vi "属性节点控制界面.vi"() -> ()   [LabVIEW 2010]
panel:
  out "执行:状态":T1(ring)
  out "前面板窗口:状态":T2(ring)
  in  "停止 3":bool
  out "数字(0-1) 3":dbl
  out "前面板窗口:在最前 2":bool
  out "数字(0-1)":dbl
  in  "布尔":bool
  out "2":dbl format="%#_11g"
  in  "停止":bool
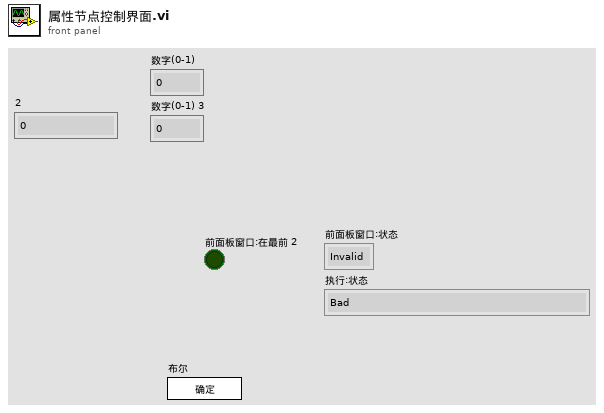
[diagram p1: front panel]
types:
  T1 = enum32{"Bad", "Idle", "Run top level", "Running"}
  T2 = enum32{"Invalid", "Standard", "Closed", "Hidden", "Minimized", "Maximized"}
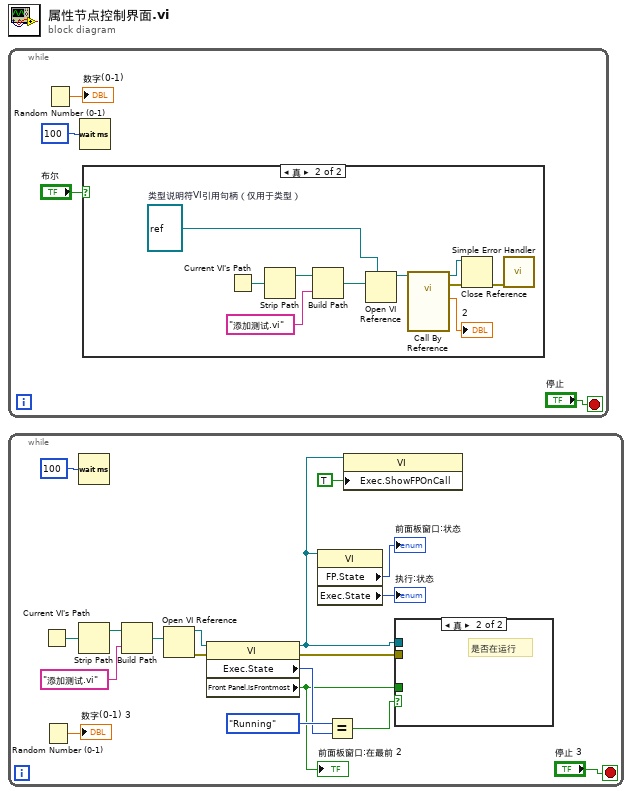
[diagram p0: block diagram]
diagram:
  n1 = while {
    stop <- "停止" stop-if-true
    n2 = Random Number (0-1)() -> (number: 0 to 1=→"数字(0-1)":dbl)
    n3 = Wait (ms)(milliseconds to wait=u32 100 ("等待时间（毫秒）")) -> ()  [unwired: 1 out]
    n4 = case shown="真" "布尔" {
      frame False {
      }
      frame True {
        w9 = refnum<vi> refnum  # 类型说明符VI引用句柄（仅用于类型）
        n5 = Current VI's Path() -> (path=w14:path)
        n6 = Strip Path(path=w14) -> (stripped path=w13:path)  [unwired: 1 out]
        n7 = Build Path(base path=w13, name or relative path="添加测试.vi" ("名称或相对路径")) -> (appended path=w11:path)
        n8 = Open VI Reference(type specifier VI Refnum (for type only)=w9, vi path=w11) -> (vi reference=w10:refnum<vi>)  [unwired: 4 in, 1 out]
        n9 = call-by-ref "?"(reference=w10) -> (reference out=w7:refnum<vi>, error out=w6:errorcluster, "手机号码"=→"2":dbl)  [unwired: 12 in]
        n10 = Close Reference(reference=w7, error in (no error)=w6) -> (error out=w5:errorcluster)
        n11 = call <vilib>:"Simple Error Handler.vi"("error in (no error)"=w5) -> ()  [unwired: 4 in, 5 out]
      }
    }
  }
  n12 = while {
    stop <- "停止 3" stop-if-true
    n13 = Current VI's Path() -> (path=w30:path)
    n14 = Random Number (0-1)() -> (number: 0 to 1=→"数字(0-1) 3":dbl)
    n15 = Wait (ms)(milliseconds to wait=u32 100 ("等待时间（毫秒）")) -> ()  [unwired: 1 out]
    n16 = Strip Path(path=w30) -> (stripped path=w22:path)  [unwired: 1 out]
    n17 = Build Path(base path=w22, name or relative path="添加测试.vi" ("名称或相对路径")) -> (appended path=w20:path)
    n18 = Open VI Reference(vi path=w20) -> (vi reference=w23:refnum<vi>, error out=w24:errorcluster)  [unwired: 5 in]
    n19 = property class="VI"(reference=w23, error in=w24) -> (reference out=w17:refnum<vi>, error out=w26:errorcluster, "Exec.State"=w27:T1, "Front Panel.IsFrontmost"=w25:bool)
    "前面板窗口:在最前 2" <- w25
    n20 = property class="VI"(reference=w17) -> ("FP.State"=→"前面板窗口:状态":T2, "Exec.State"=→"执行:状态":T1)  [unwired: 1 in, 2 out]
    n21 = Equal?(x=T1."Running", y=w27) -> (x = y?=w29:bool)
    n22 = property class="VI"(reference=w17, "Exec.ShowFPOnCall"=TRUE ("执行:调用时显示前面板")) -> ()  [unwired: 1 in, 2 out]
    n23 = case shown="真" w29 {
      tunnel: w25 -> [_ _]
      tunnel: w17 -> [_ _]
      tunnel: w26 -> [_ _]
      frame False {
      }
      frame True {
        # "是否在运行"
      }
    }
  }
